vi "Pozycjonuje Obiekty Konfiguracja.vi"(8 "error in (no error)":errorcluster, 10 "Kwadratowy":T1[](array[typedef]), 11 "Array in":refnum<vi>[](array[refnum])) -> (0 "error out":errorcluster)   [LabVIEW 2014]
doc: "Ustawia położenie w zakładce Konfiguracja obiektów:\nPrzemieszczenie\nRejestracja Szybka\nKanały cyfrowe\nRejestracja Wolna"
uses:
  <vilib>/Utility/miscctls.llb/LVPositionTypeDef.ctl
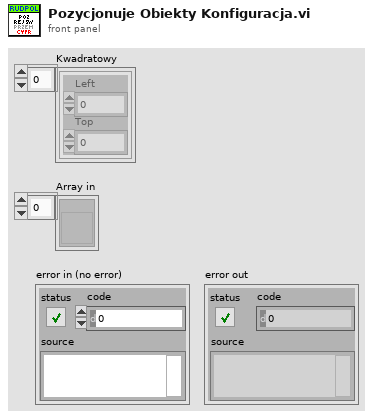
[diagram p1: front panel]
types:
  T1 = typedef "LVPositionTypeDef.ctl" = cluster{"Left":i32, "Top":i32}
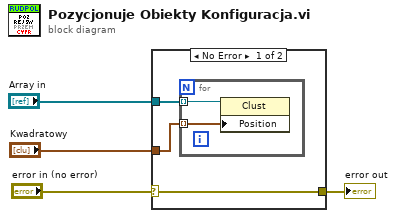
[diagram p0: block diagram]
diagram:
  n1 = case shown="No Error" "error in (no error)" {
    selector: "error in (no error)" -> [w5 w10]
    tunnel: "Kwadratowy" -> [w7 _]
    tunnel: "Array in" -> [w6 _]
    tunnel: [w5 w10] -> w1
    frame No Error {
      n2 = for {
        tunnel: w6 -> [w9] mode=indexing
        tunnel: w7 -> [w8] mode=indexing
        n3 = property class="Clust"(reference=w9, "Position"=w8) -> ()  [unwired: 1 in, 2 out]
      }
    }
    frame Error {
    }
  }
  "error out" <- w1
